vi "U8BitJoin.vi"(1 "array":u8[](array[numeric])=[0, 0, 0], 2 "hi":u8) -> (0 "U32":u32 format="%032b")   [LabVIEW 2014]
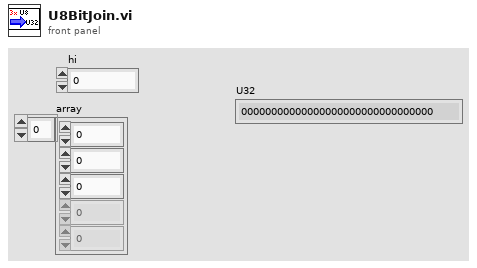
[diagram p1: front panel]
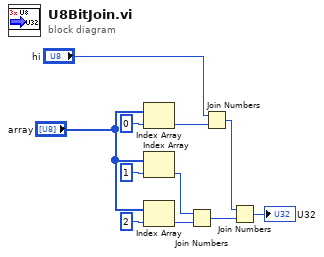
[diagram p0: block diagram]
diagram:
  n1 = Index Array(array="array", index=0) -> (element=w10:u8)
  n2 = Index Array(array="array", index=1) -> (element=w6:u8)
  n3 = Index Array(array="array", index=2) -> (element=w5:u8)
  n4 = Join Numbers(hi=w6, lo=w5) -> ((hi.lo)=w4:u16)
  n5 = Join Numbers(hi="hi", lo=w10) -> ((hi.lo)=w3:u16)
  n6 = Join Numbers(hi=w3, lo=w4) -> ((hi.lo)=→"U32":u32)
